vi "QSI Get System Default Printer.vi"(3 "error in (no error)":errorcluster) -> (0 "error out":errorcluster, 2 "System Default Printer":string)   [LabVIEW 2015]
doc: "This VI returns the current system default printer.\n\nProgrammer: Quentin Alldredge\n<b> </b> <b> </b>\n©2013, Q Software Innovations, LLC.\n\nWritten in National Instruments LabVIEW™ 2013.\n\nAuthored by Quentin Alldredge\nQ@qsoftwareinnovations.com\nwww.qsoftwareinnovations.com\n\nAll rights reserved."
uses:
  <vilib>/registry/registry.llb/Registry RtKey.ctl
  <vilib>/registry/registry.llb/Read Registry Value Simple STR.vi
panel:
  # "Input"
  # "Output"
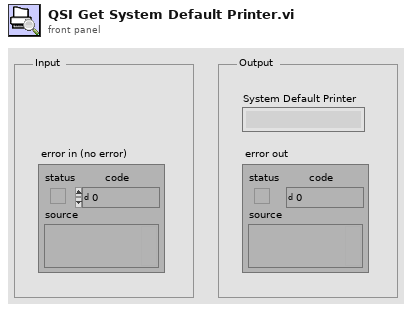
[diagram p1: front panel]
types:
  T1 = typedef "Registry RtKey.ctl" = enum32{"HKEY_CLASSES_ROOT", "HKEY_CURRENT_USER", "HKEY_LOCAL_MACHINE", "HKEY_USERS", "HKEY_PERFORMANCE_DATA", "HKEY_CURRENT_CONFIG", "HKEY_DYN_DATA"}
  T2 = typedef "Registry refnum.ctl" = refnum<k1>
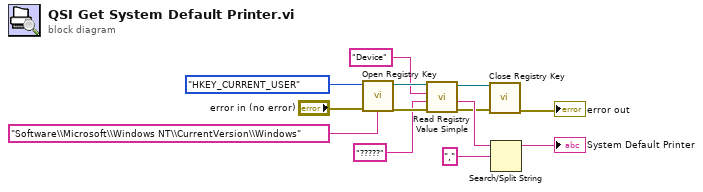
[diagram p0: block diagram]
diagram:
  n1 = call <vilib>:"Open Registry Key.vi"("error in (no error)"="error in (no error)", "subkey"="Software\\Microsoft\\Windows NT\\CurrentVersion\\Windows", "root key (HKEY_LOCAL_MACHINE)"=Registry_RtKey."HKEY_CURRENT_USER") -> ("error out"=w10:errorcluster, "refnum out"=w11:T2)  [unwired: 7 in]
  n2 = call-poly <vilib>:"Read Registry Value Simple.vi"("error in (no error)"=w10, "default data"="?????", "value"="Device", "refnum"=w11) -> ("error out"=w1:errorcluster, "String/Binary data"=w7:string, "refnum out"=w2:T2)  [unwired: 2 in, 1 out]
  n3 = call <vilib>:"Close Registry Key.vi"("error in (no error)"=w1, "refnum"=w2) -> ("error out"=→"error out":errorcluster)  [unwired: 5 in]
  n4 = Search/Split String(string=w7, search string/char (-)=",") -> (substring before match=→"System Default Printer":string)  [unwired: 1 in, 2 out]
